vi "NTJ_Srv_Bld_Msg_18.vi"(10 "Field ID":T1, 11 "Field Value Out":T2) -> (3 "Msg Buffer":string)   [LabVIEW 2019]
uses:
  <vilib>/Rock Robotics/Network Tables/Field Data.ctl
  <vilib>/Rock Robotics/Network Tables/Field Type.ctl
  <vilib>/Rock Robotics/Network Tables/Sequence.ctl
  <vilib>/Rock Robotics/Network Tables/Field ID.ctl
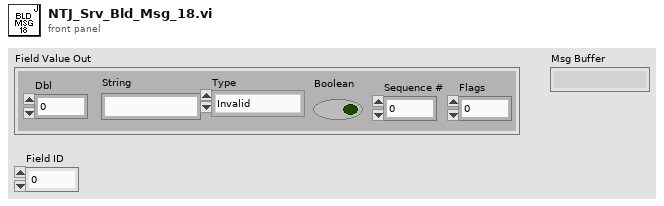
[diagram p1: front panel]
types:
  T1 = typedef "Field ID.ctl" = i32
  T2 = typedef "Field Data.ctl" = cluster{"Dbl":dbl, "String":string, "Type":T3, "Boolean":bool, "Sequence #":T4, "Flags":u8}
  T3 = typedef "Field Type.ctl" = enum8{"Invalid", "Bool", "Numeric", "String", "Raw", "Boolean Array", "Numeric Array", "String Array", "RPC"}
  T4 = typedef "Sequence.ctl" = u16
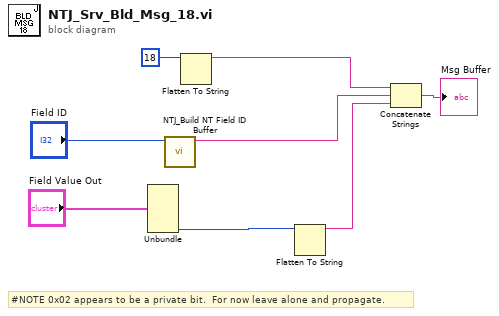
[diagram p0: block diagram]
diagram:
  # "#NOTE 0x02 appears to be a private bit.  For now leave alone and propagate."
  n1 = Unbundle("Field Value Out") -> ("Flags"=w1:u8)  [unwired: 5 out]
  n2 = call "NTJ_Build NT Field ID Buffer.vi"("Field ID"="Field ID") -> ("Data Buffer"=w6:string)  [unwired: 10 in]
  n3 = Flatten To String(anything=u8 18 ("bytes to read")) -> (data string=w5:string)  [unwired: 3 in, 2 out]
  n4 = Flatten To String(anything=w1) -> (data string=w8:string)  [unwired: 3 in, 2 out]
  n5 = Concatenate Strings(w5, w6, w8) -> (→"Msg Buffer":string)
